vi "Find Channel.vi"(0 "Strings And Values []":cluster{"String":string, "Value":u8}[](array[cluster]), 7 "Value":u8) -> (8 "Channel":string)   [LabVIEW 2010]
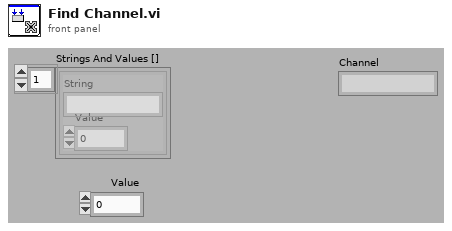
[diagram p1: front panel]
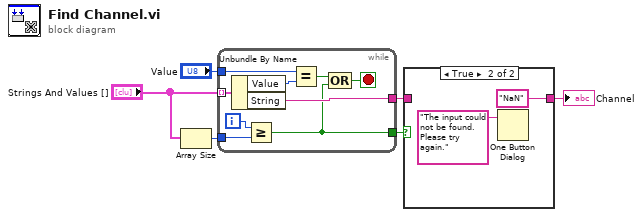
[diagram p0: block diagram]
diagram:
  n1 = Array Size(array="Strings And Values []") -> (size(s)=w4:i32)
  n2 = while {
    tunnel: "Strings And Values []" -> [w15] mode=indexing
    tunnel: "Value" -> [w13]
    tunnel: [w12] -> w2
    tunnel: w4 -> [w8]
    tunnel: [w7] -> w3
    i -> [w9]
    stop <- w10 stop-if-true
    n3 = Unbundle By Name(w15) -> ("Value"=w14:u8, "String"=w12:string)
    n4 = Greater Or Equal?(x=w9, y=w8) -> (x >= y?=w7:bool)
    n5 = Equal?(x=w13, y=w14) -> (x = y?=w11:bool)
    n6 = Compound Arithmetic op=OR(w11, w7) -> (w10:bool)
  }
  n7 = case shown="TRUE" w3 {
    tunnel: w2 -> [w16 _]
    tunnel: [w16 "NaN" ("String")] -> w1
    frame False {
    }
    frame True {
      n8 = One Button Dialog(message="The input could not be found.  Please try again.") -> ()  [unwired: 2 out]
    }
  }
  "Channel" <- w1
